vi "Make String Mermaid Safe.vi"(11 "Source CSM":string) -> (3 "result string":string)   [LabVIEW 2020]
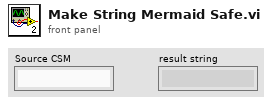
[diagram p1: front panel]
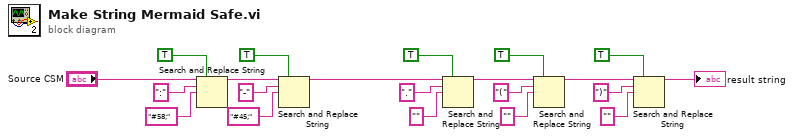
[diagram p0: block diagram]
diagram:
  n1 = Search and Replace String(replace all?=TRUE ("replace all? (F)"), input string="Source CSM", search string=":", replace string="#58;" ("search string")) -> (result string=w14:string)  [unwired: 4 in, 3 out]
  n2 = Search and Replace String(replace all?=TRUE ("replace all? (F)"), input string=w14, search string="-", replace string="#45;" ("search string")) -> (result string=w6:string)  [unwired: 4 in, 3 out]
  n3 = Search and Replace String(replace all?=TRUE ("replace all? (F)"), input string=w6, search string=".", replace string="" ("search string")) -> (result string=w13:string)  [unwired: 4 in, 3 out]
  n4 = Search and Replace String(replace all?=TRUE ("replace all? (F)"), input string=w13, search string="(", replace string="" ("search string")) -> (result string=w2:string)  [unwired: 4 in, 3 out]
  n5 = Search and Replace String(replace all?=TRUE ("replace all? (F)"), input string=w2, search string=")", replace string="" ("search string")) -> (result string=→"result string":string)  [unwired: 4 in, 3 out]
